vi "摆臂角度读取-子.vi"(1 "error in":errorcluster caption="错误输入", 2 "task/channels in":refnum<k21> caption="任务/通道输入") -> (0 "摆臂角度输出":dbl)   [LabVIEW 2015]
uses:
  <vilib>/DAQmx/read.llb/DAQmx Read (Counter U32 1Chan 1Samp).vi
  <vilib>/DAQmx/miscellaneous.llb/DAQmx Fill In Error Info.vi
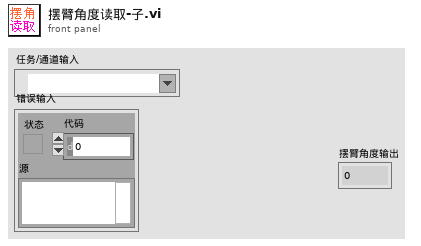
[diagram p1: front panel]
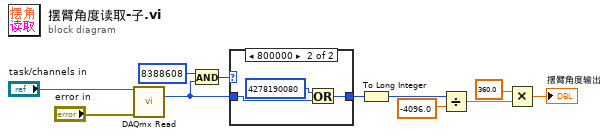
[diagram p0: block diagram]
diagram:
  n1 = call-poly <vilib>:"DAQmx Read.vi"("task/channels in"="task/channels in", "error in"="error in") -> ("data"=w9:u32)  [unwired: 11 in, 2 out]
  n2 = And(x=u32 8388608, y=w9) -> (x .and. y?=w11:u32)
  n3 = case shown="800000" w11 {
    tunnel: w9 -> [w12 w15]
    tunnel: [w12 w14] -> w8
    frame 0, Default {
    }
    frame 8388608 {
      n4 = Or(x=u32 4278190080, y=w15) -> (x .or. y?=w14:u32)
    }
  }
  n5 = To Long Integer(number=w8) -> (32bit integer=w3:i32)
  n6 = Divide(x=w3, y=-4096.0) -> (x/y=w6:dbl)
  n7 = Multiply(x=360.0, y=w6) -> (x*y=→"摆臂角度输出":dbl)
